vi "SVFA Frequency Response (1x1) (Mag-Phase).vi"(0 "stimulus signal X [EUx]":waveform(dbl), 1 "response signal Y [EUy]":waveform(dbl), 2 "window":T8=1 items=["None"=0, "Hanning"=1, "Hamming"=2, "Blackman-Harris"=3, "Exact Blackman"=4, "Blackman"=5, "Flat Top"=6, "4 Term B-Harris "=7, "7 Term B-Harris"=8, "Low Sidelobe"=9, "Force - Exponential"=10, "Blackman Nuttall"=11, "Triangle"=30, "Bartlett-Hanning"=31, "Bohman"=32, "Parzen"=33, "Welch"=34, "Kaiser"=60, "Dolph-Chebyshev"=61, "Gaussian"=62], 4 "view":T10={"dB On (T)"=TRUE, "unwrap phase (F)"=FALSE, "convert to degree (T)"=TRUE}, 5 "error in (no error)":errorcluster, 6 "FRF mode":enum16{"H1", "H2", "H3"}(ring), 7 "averaging parameters":T9={"averaging mode"=enum."No averaging", "weighting mode"=enum."Exponential", "number of averages"=10, "linear mode"=enum."One shot"}, 8 "force/exp settings":T7={"force window [%]"=50.0, "exp window [%]"=10.0} {"exp window [%]" min=0.0 max=100.0 format="%.2f"; "force window [%]" min=0.0 max=100.0 format="%.2f"}, 9 "restart averaging (F)":bool) -> (11 "averaging done":bool, 12 "coherence":cluster{"f0":dbl, "df":dbl, "coherence":dbl[]} {"coherence" format="%.2f"; "df" format="%.2f"; "f0" format="%.2f"}, 13 "averages completed":dbl, 14 "magnitude [dB EUy/EUx]":cluster{"f0":dbl, "df":dbl, "magnitude":dbl[]} {"magnitude" format="%.2p"; "df" format="%.2p"; "f0" format="%.2p"}, 15 "magnitude unit label":string, 16 "phase [degrees]":cluster{"f0":dbl, "df":dbl, "phase":dbl[]} {"phase" format="%.2f"; "df" format="%.2f"; "f0" format="%.2f"}, 17 "phase unit label":string, 18 "spectrum info":T1={"channel name"="", "description"="", "x-axis units"=0, "spectral info"={"spectrum type"=enum."Power [Magnitude^2]", "linear/dB"=enum."linear", "window"=0, "window size"=0, "FFT size"=0}, "engineering units"=0, "custom label"="", "dB reference [EU]"=0.0, "peak units"=enum."rms", "weighting filter"=0, "spectral density?"=FALSE, "unit label"="", "spectrum skewed?"=FALSE, "complimentary spectrum units"=enum."none"} {"x-axis units" items=["Time (s)"=0, "Frequency-CB (Hz)"=1, "Frequency-CPB (Hz)"=1248, "Frequency-Arbitrary (Hz)"=2357, "Quefrency (s)"=2, "Revolutions (rev)"=3, "Order"=4, "Speed (RPM)"=11, "Speed (rad/s)"=21, "Index"=65535]; "weighting filter" items=["Linear", "A-weighting", "B-weighting", "C-weighting", "ITU-R 468-4", "Dolby", "CCITT", "C-message", "Wb", "Wc", "Wd", "We", "Wf", "Wh", "Wj", "Wk", "Wm", "AES17 20 kHz lowpass", "AES17 40 kHz lowpass", "AES17 20 kHz highpass", "AES17 40 kHz highpass"]; "dB reference [EU]" format="%.2f"; "engineering units" items=["custom..."=0, "V"=1, "A"=21, "C"=30, "pC"=31, "s"=32, "-"=29, "Pa"=2, "N"=20, "g"=3, "m/s^2"=4, "m/s"=5, "m"=6, "mm/s"=12, "mm"=13, "micron/s"=14, "micron"=15, "in/s^2"=7, "in/s"=8, "in"=9, "mil/s"=10, "mil"=11, "rad/s^2"=16, "rad/s"=17, "rad"=18, "deg/s^2"=26, "deg/s"=27, "deg"=28, "RPM"=22, "cycle/s^2"=23, "Hz"=24, "cycle"=25, "strain"=19]; "spectral info"."window" items=["None "=0, "Hanning"=1, "Hamming"=2, "Blackman-Harris"=3, "Exact Blackman"=4, "Blackman"=5, "Flat Top"=6, "4 Term B-Harris "=7, "7 Term B-Harris"=8, "Low Sidelobe"=9, "Force - Exponential"=10, "Gaussian"=62]}, 19 "error out":errorcluster)   [LabVIEW 2017]
doc: "Computes the magnitude, phase, and coherence of the frequency response of the device under test [DUT]. This VI computes the ratio of the output to the input of the DUT. Wire data to the <B>stimulus signal X [Eux]</B> and <B>response signal Y [Euy]</B> inputs to determine the polymorphic instance to use or manually select the instance."
uses:
  <vilib>/addons/_NISVFA/_Shared subVIs/Controls/svc_Window [Dual FFT].ctl
  <vilib>/addons/_NISVFA/_Shared subVIs/Controls/svc_Spectrum Info.ctl
  <vilib>/addons/_NISVFA/_Shared subVIs/Controls/svc_X-Axis Units.ctl
  <vilib>/addons/_NISVFA/_Shared subVIs/Controls/svc_Spectrum Type.ctl
  <vilib>/addons/_NISVFA/_Shared subVIs/Controls/svc_Engineering Units Text Ring.ctl
  <vilib>/addons/_NISVFA/_Shared subVIs/Controls/svc_Weighting Filter Text Ring.ctl
  <vilib>/addons/_NISVFA/_Shared subVIs/Controls/svc_Complimentary Spectrum Units.ctl
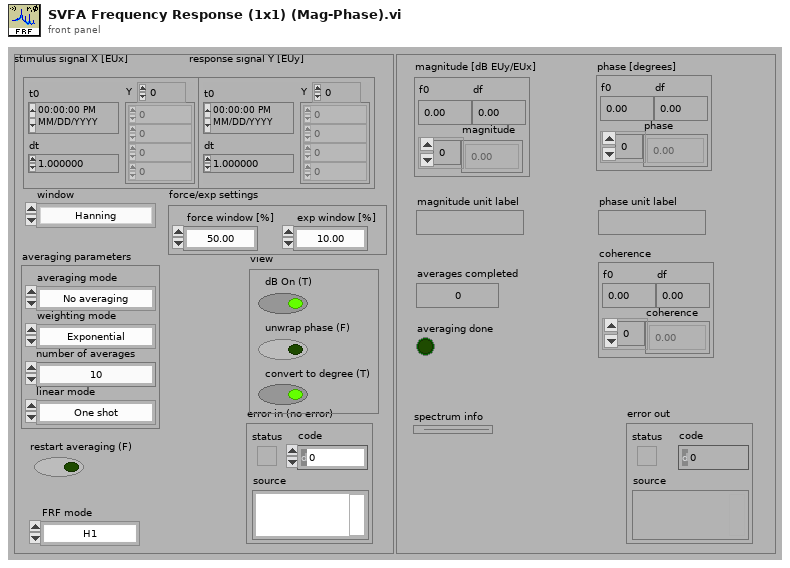
[diagram p1: front panel]
types:
  T1 = typedef "svc_Spectrum Info.ctl" = cluster{"channel name":string, "description":string, "x-axis units":T2, "spectral info":cluster{"spectrum type":T3, "linear/dB":enum16{"linear", "dB"}, "window":u16, "window size":i32, "FFT size":i32}, "engineering units":T4, "custom label":string, "dB reference [EU]":dbl, "peak units":enum16{"rms", "peak", "peak-peak"}, "weighting filter":T5, "spectral density?":bool, "unit label":string, "spectrum skewed?":bool, "complimentary spectrum units":T6}
  T2 = typedef "svc_X-Axis Units.ctl" = u16
  T3 = typedef "svc_Spectrum Type.ctl" = enum16{"FFT Spectrum [complex]", "Amplitude [Magnitude]", "Power [Magnitude^2]", "Cross Spectrum [complex]", "Frequency Response [Complex]"}
  T4 = typedef "svc_Engineering Units Text Ring.ctl" = u16
  T5 = typedef "svc_Weighting Filter Text Ring.ctl" = u16
  T6 = typedef "svc_Complimentary Spectrum Units.ctl" = enum16{"none", "radians", "degrees", "cycles", "imaginary"}
  T7 = cluster{"force window [%]":dbl, "exp window [%]":dbl}
  T8 = typedef "svc_Window [Dual FFT].ctl" = u32
  T9 = cluster{"averaging mode":enum16{"No averaging", "Vector averaging", "RMS averaging", "Peak hold"}, "weighting mode":enum16{"Linear", "Exponential"}, "number of averages":u32, "linear mode":enum16{"One shot", "Auto restart"}}
  T10 = cluster{"dB On (T)":bool, "unwrap phase (F)":bool, "convert to degree (T)":bool}
  T11 = enum16{"Cross spectrum", "Frequency response", "Coherent output power"}
  T12 = enum16{"Restart processing", "Continue processing", "Skip processing"}
  T13 = cluster{"f0":dbl, "df":dbl, "complex spectrum":cdb[]}
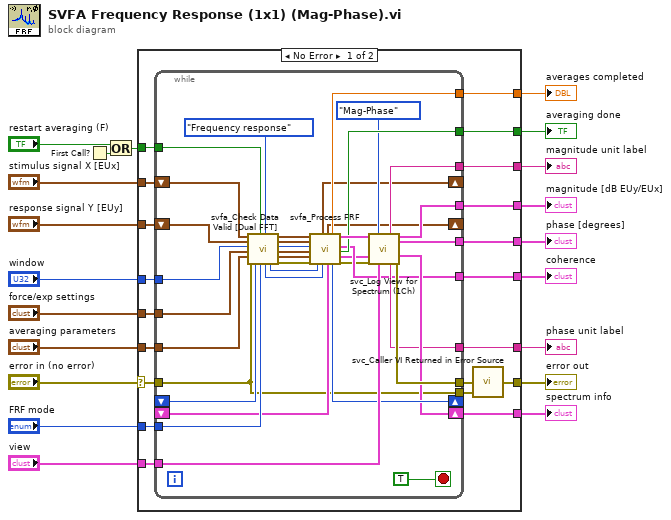
[diagram p0: block diagram]
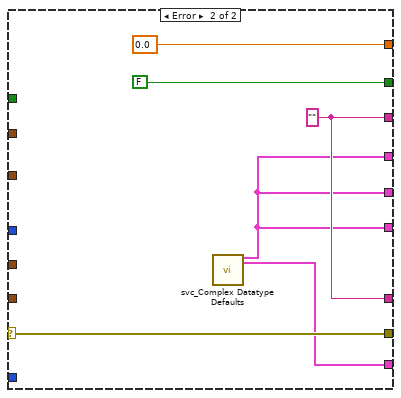
[diagram p2: hidden frame]
diagram:
  n1 = First Call?() -> (First Call?: T/F=w3:bool)
  n2 = Or(x="restart averaging (F)", y=w3) -> (x .or. y?=w2:bool)
  n3 = case shown="No Error" "error in (no error)" {
    selector: "error in (no error)" -> [w40 w83]
    tunnel: "averaging parameters" -> [w29 _]
    tunnel: "window" -> [w30 _]
    tunnel: "force/exp settings" -> [w28 _]
    tunnel: "stimulus signal X [EUx]" -> [w39 _]
    tunnel: "response signal Y [EUy]" -> [w38 _]
    tunnel: [w35 w79] -> w14
    tunnel: [w34 w79] -> w13
    tunnel: [w32 w79] -> w12
    tunnel: [w22 w83] -> w11
    tunnel: [w37 FALSE ("averaging done")] -> w10
    tunnel: [w36 0.0 ("averages completed")] -> w9
    tunnel: w2 -> [w23 _]
    tunnel: "view" -> [w31 _]
    tunnel: "FRF mode" -> [w27 _]
    tunnel: [w26 w78] -> w6
    tunnel: [w25 w80] -> w5
    tunnel: [w24 w80] -> w4
    frame No Error {
      n4 = while {
        tunnel: w23 -> [w53]
        tunnel: [w55] -> w24
        tunnel: [w56] -> w25
        shift-left: _ -> [w54]
        shift-right: [w59] -> _
        tunnel: w27 -> [w51]
        tunnel: w28 -> [w69]
        tunnel: w29 -> [w67]
        tunnel: w30 -> [w70]
        tunnel: w31 -> [w71]
        tunnel: [w48] -> w32
        tunnel: [w72] -> w33
        tunnel: [w46] -> w34
        tunnel: [w73] -> w35
        tunnel: [w75] -> w36
        tunnel: [w58] -> w37
        tunnel: w40 -> [w41]
        shift-right: [w57] -> w26
        shift-left: _ -> [w44]
        shift-right: [w43] -> _
        shift-left: w39 -> [w77]
        shift-right: [w42] -> _
        shift-left: w38 -> [w76]
        tunnel: [w41] -> w21
        stop <- TRUE stop-if-true
        n5 = call <vilib>:"svfa_Check Data Valid [Dual FFT].vi"("stimulus [X]"=w77, "response [Y]"=w76, "window"=w70, "force/exp settings"=w69, "averaging parameters"=w67, "error in (no error)"=w41, "processing control in"=w54, "restart averaging (F)"=w53, "FRF mode"=w51, "measurement"=T11."Frequency response") -> ("dup FRF mode"=w50:enum16{"H1", "H2", "H3"}, "processing control out"=w60:T12, "dup stimulus [X]"=w66:waveform(dbl), "dup response [Y]"=w65:waveform(dbl), "window"=w64:T8, "dup force/exp settings"=w63:T7, "dup averaging parameters"=w62:T9, "error out"=w61:errorcluster)  [unwired: 2 in]
        n6 = call <vilib>:"svfa_Process FRF.vi"("stimulus signal X [EUx]"=w66, "response signal Y [EUy]"=w65, "window"=w64, "force/exp settings"=w63, "averaging parameters"=w62, "error in (no error)"=w61, "processing control"=w60, "FRF mode"=w50, "spectrum info in"=w44) -> ("stimulus signal X [EUx]"=w43:waveform(dbl), "response signal Y [EUy]"=w42:waveform(dbl), "averages completed"=w75:dbl, "processing control"=w59:T12, "complex frequency response"=w74:T13, "coherence"=w48:cluster{"f0":dbl, "df":dbl, "coherence":dbl[]}, "averaging done"=w58:bool, "spectrum info out"=w45:T1, "error out"=w47:errorcluster)  [unwired: 2 in]
        n7 = call <vilib>:"svc_Log View for Spectrum (1Ch).vi"("complex spectrum"=w74, "View"=enum16{"Mag-Phase", "Real-Imaginary"}."Mag-Phase", "spectrum info in"=w45, "error in (no error)"=w47, "view"=w71) -> ("unit label [mag or real]"=w56:string, "magnitude or real"=w73:cluster{"f0":dbl, "df":dbl, dbl[]}, "phase or imag"=w46:cluster{"f0":dbl, "df":dbl, dbl[]}, "spectrum info out"=w57:T1, "unit label [phase or imag]"=w55:string, "error out"=w72:errorcluster)  [unwired: 5 in]
      }
      n8 = call <vilib>:"svc_Caller VI Returned in Error Source.vi"("warning input to caller"=w21, "error in (no error)"=w33) -> ("error out"=w22:errorcluster)  [unwired: 3 in]
    }
    frame Error {
      w80 = "" ("unit label (mag or real)")
      n9 = call <vilib>:"svc_Complex Datatype Defaults.vi"() -> ("empty spectrum"=w79:cluster{"f0":dbl, "df":dbl, "magnitude":dbl[]}, "dead spectrum info"=w78:T1)  [unwired: 11 in, 7 out]
    }
  }
  "error out" <- w11
  "magnitude [dB EUy/EUx]" <- w14
  "phase [degrees]" <- w13
  "averaging done" <- w10
  "averages completed" <- w9
  "coherence" <- w12
  "spectrum info" <- w6
  "phase unit label" <- w4
  "magnitude unit label" <- w5
